vi "Table_ScrollaBar.vi"(3 "error in":errorcluster, 4 "Line to focus":string, 5 "reference in":refnum<vi>) -> (0 "error out":errorcluster, 1 "OK?":bool, 2 "reference out":refnum<vi>)   [LabVIEW 2017]
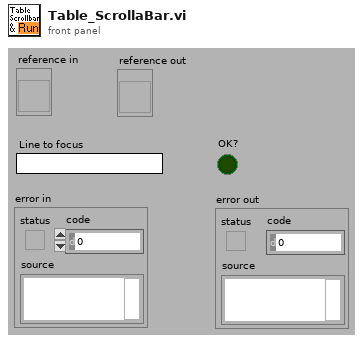
[diagram p1: front panel]
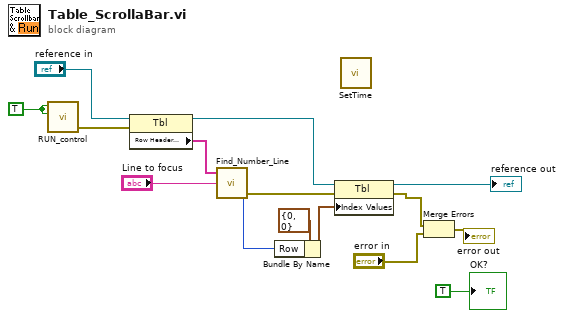
[diagram p0: block diagram]
diagram:
  w1 = TRUE ("Blinking")
  n1 = call "RUN_control.vi"("Blinking(:T)"=w1, "Value (:T)"=w1) -> ("error out"=w2:errorcluster)  [unwired: 3 in, 2 out]
  n2 = property on="Property Node" class="Tbl"(reference="reference in", error in=w2) -> (reference out=w4:refnum<vi>, "Row Header Strings[]"=w3:string[])  [unwired: 1 out]
  n3 = call "Find_Number_Line.vi"("Test Paragraph"="Line to focus", "Row Headers[]"=w3) -> ("error out"=w11:errorcluster, "Line number"=w13:i32)  [unwired: 1 in, 1 out]
  n4 = Bundle By Name(cluster=cluster{"Row":i32, "Column":i32} {"Row"=0, "Column"=0} ("Edit Position"), "Row"=w13) -> (w14:cluster{"Row":i32, "Column":i32})
  n5 = property on="Property Node" class="Tbl"(reference=w4, error in=w11, "Index Values"=w14) -> (reference out=→"reference out":refnum<vi>, error out=w7:errorcluster)
  n6 = call "SetTime.vi"() -> ()  [unwired: 11 in, 1 out]
  n7 = Merge Errors(w7, "error in") -> (→"error out":errorcluster)
  "OK?" <- TRUE ("OK?")
